vi "EnergyMonitoring.vi"() -> ()   [LabVIEW 2017]
uses:
  <vilib>/drjdpowell/SQLite Library/SQL Statement/SQL Statement.lvclass/SQL Statement.ctl
  <vilib>/drjdpowell/SQLite Library/SQL Connection/Open (path).vi
  <vilib>/drjdpowell/SQLite Library/SQL Statement/Column I64.vi
  <vilib>/drjdpowell/SQLite Library/SQL Statement/Column DBL.vi
  <vilib>/drjdpowell/SQLite Library/SQL Connection/Open (string).vi
  <vilib>/drjdpowell/SQLite Library/SQL Statement/Column Type.vi
  <vilib>/AdvancedString/Path To Command Line String.vi
  <vilib>/drjdpowell/SQLite Library/SQL Connection/Execute SQL.vi
  <vilib>/drjdpowell/SQLite Library/SQL Statement/Error Message.vi
  <vilib>/drjdpowell/SQLite Library/SQL Statement/Column Timestamp.vi
  <vilib>/drjdpowell/SQLite Library/SQL Statement/Column String.vi
  <vilib>/drjdpowell/SQLite Library/SQL Connection/Connection.lvclass
  <vilib>/drjdpowell/SQLite Library/SQL Statement/SQL Statement.lvclass
  <vilib>/drjdpowell/SQLite Library/SQLite.lvlib
panel:
  in  "Tab Control":enum32{"Monitor Values", "Monitor Diagram"}(tab)
  in  "Update":bool
  in  "Monitor Data of the Element":i32(listbox)=-1
  in  "Count of Points":i64(slide)=50 scale=0.0..100.0
  in  "x - Axis":u16(ring) items=["Index"]
  in  "y - Axis":i32(listbox)
  out "Graph":cluster{dbl[], dbl[]}(graph) caption="Selected data points (greater than \"minimum\")"
  in  "Update Trigger [sec]":i32=3
  in  "Count of Points Diagram":i64(slide)=50 scale=0.0..100.0
  out "Column:Get Column I64":i64
  in  "Field Elements":i32(listbox)
  in  "stop":bool
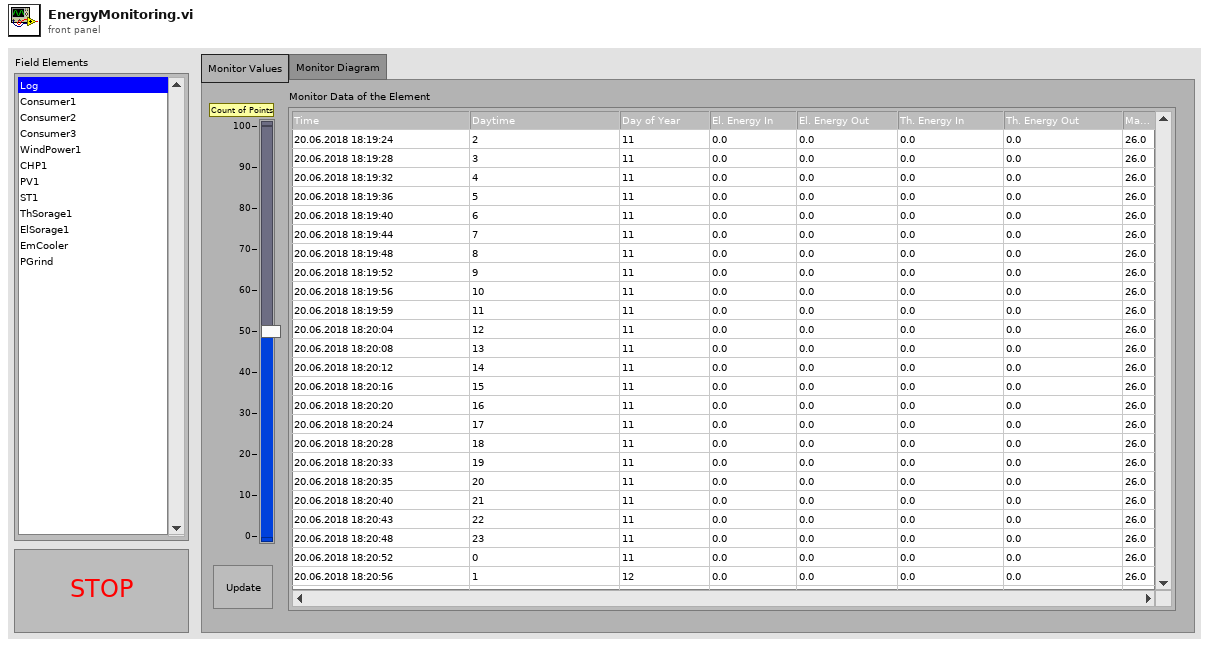
[diagram p1: front panel]
types:
  T1 = enum16{"New or existing", "Existing", "Read only"}
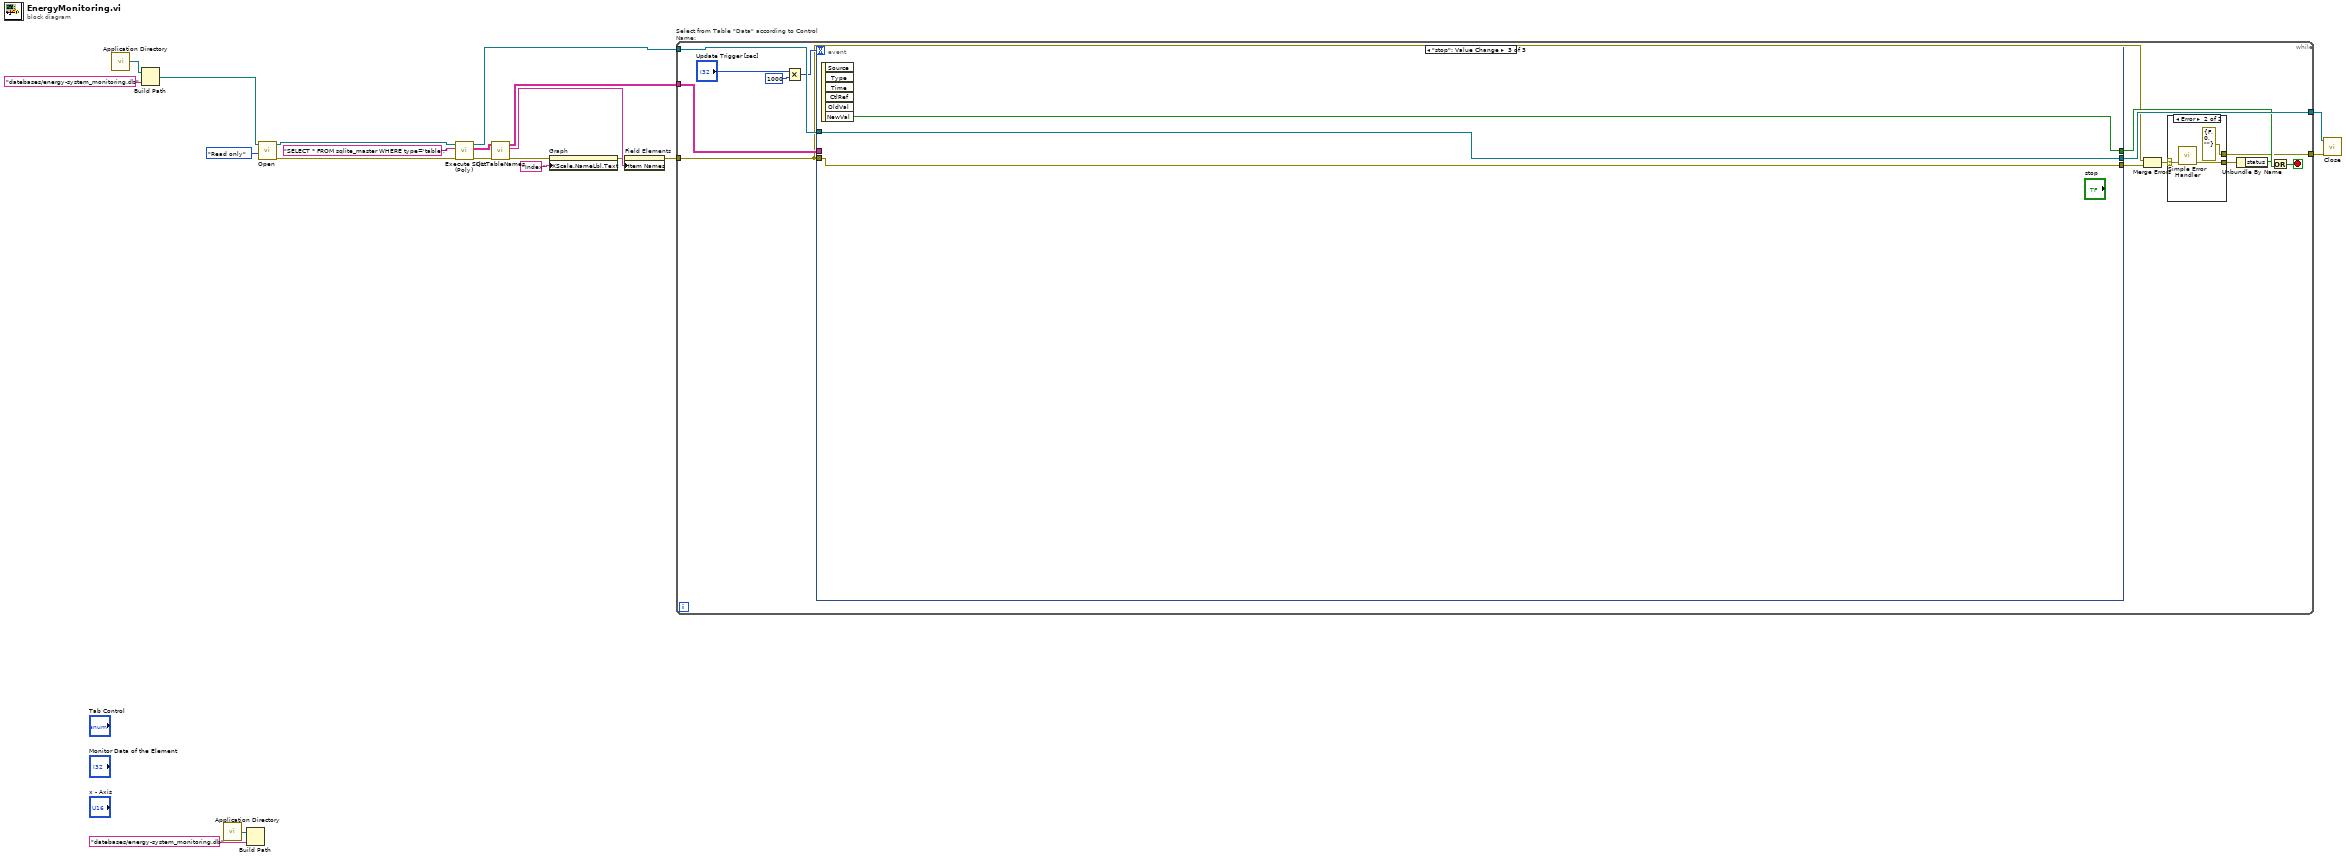
[diagram p0: block diagram]
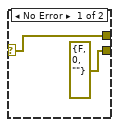
[diagram p2: hidden frame]
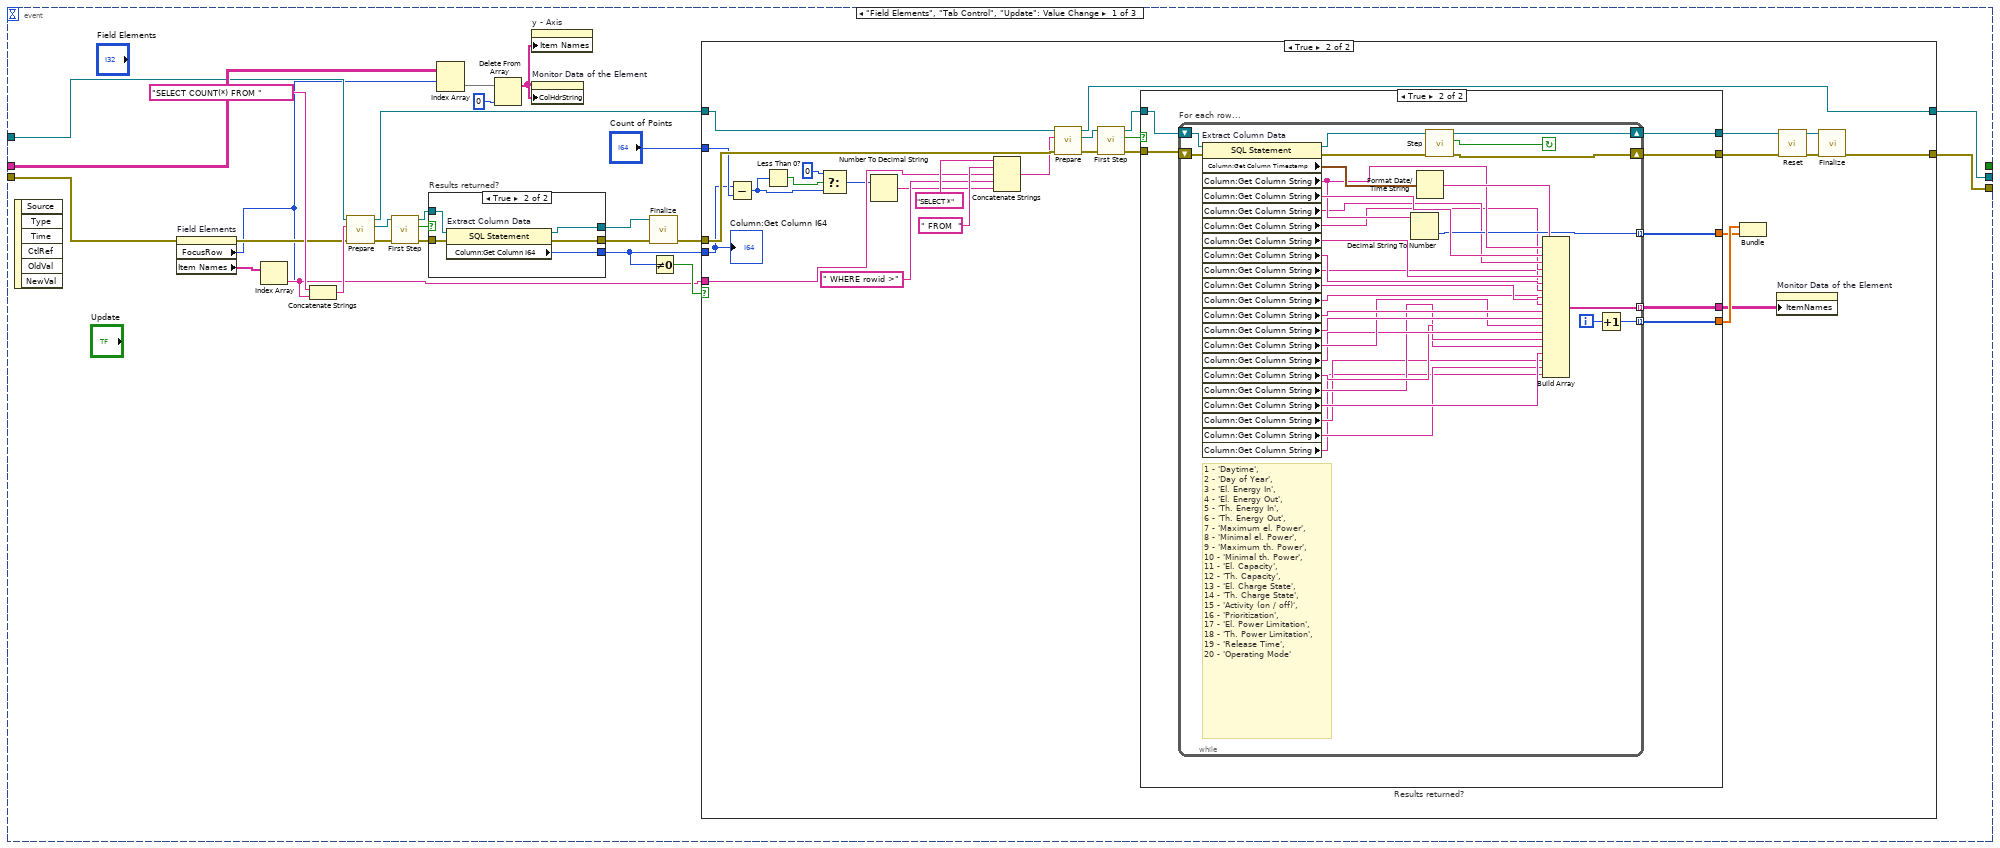
[diagram p3: hidden frame]
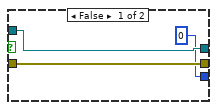
[diagram p4: hidden frame]
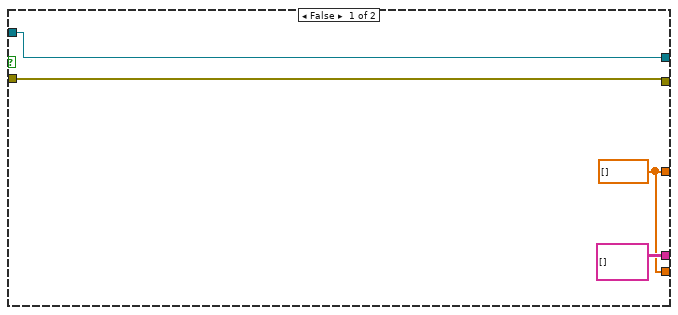
[diagram p6: hidden frame]
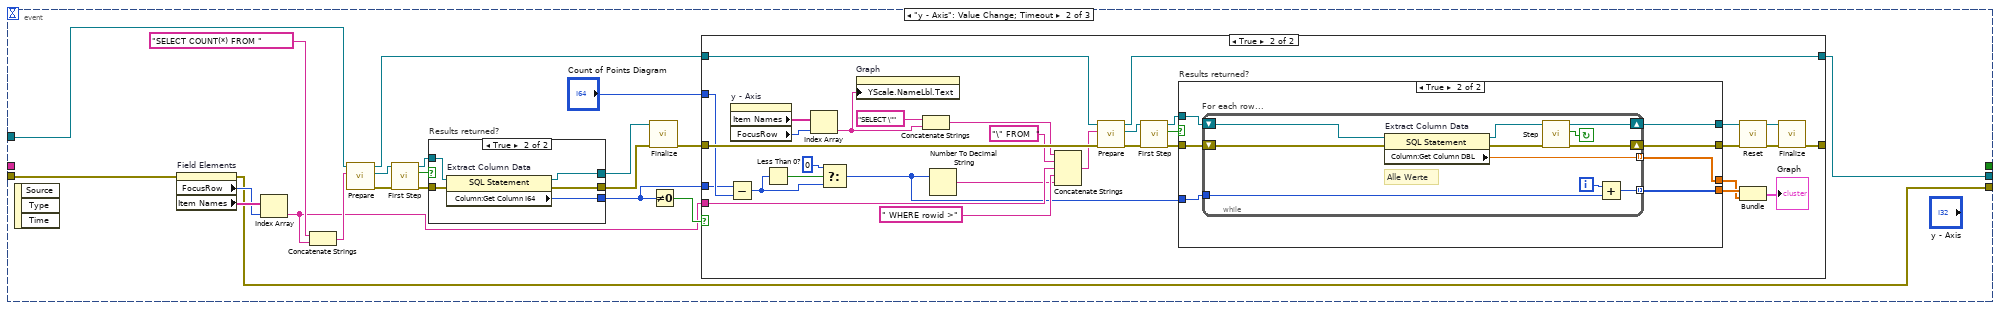
[diagram p7: hidden frame]
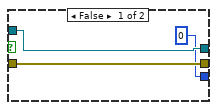
[diagram p8: hidden frame]
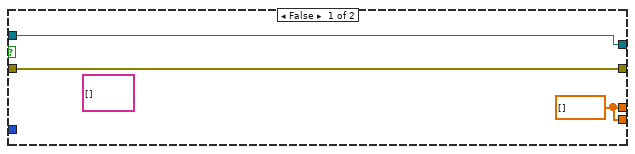
[diagram p10: hidden frame]
diagram:
  n1 = call <vilib>:"Application Directory.vi"() -> ("Application Directory"=w3:path)
  n2 = Build Path(base path=w3, name or relative path="datebases/energy-system_monitoring.db" ("Name oder relativer Pfad")) -> (appended path=w1:path)
  n3 = call <vilib>:"Application Directory.vi"() -> ("Application Directory"=w18:path)
  n4 = Build Path(base path=w18, name or relative path="datebases/energy-system_monitoring.db" ("Name oder relativer Pfad")) -> ()  [unwired: 1 out]
  n5 = call-poly <vilib>:"Open.vi"("File Option"=T1."Read only", "db file"=w1) -> ("error out"=w17:errorcluster, "SQLite Connection out"=w16:refnum<class "Connection.lvclass">)  [unwired: 8 in]
  n6 = call-poly <vilib>:"Execute SQL (Poly).vi"("error in (no error)"=w17, "SQL"="SELECT * FROM sqlite_master WHERE type='table';" ("String"), "SQLite Connection in"=w16) -> ("error out"=w6:errorcluster, "Result Set"=w10:string[][], "SQLite Connection out"=w14:refnum<class "Connection.lvclass">)  [unwired: 5 in, 1 out]
  n7 = call "ListTableNames.vi"("error in (no error)"=w6, "Result Set"=w10) -> ("error out"=w5:errorcluster, "Table Names"=w9:string[], "List of Tabel and Column Names"=w8:string[][])  [unwired: 7 in]
  n8 = property on="Graph" class="XYGraph (strict)"(error in=w5, "XScale.NameLbl.Text"="Index" ("X Scale.Name Label.Text")) -> (error out=w4:errorcluster)  [unwired: 1 in, 1 out]
  n9 = property on="Field Elements" class="LstBox (strict)"(error in=w4, "Item Names"=w9) -> (error out=w15:errorcluster)  [unwired: 1 in, 1 out]
  n10 = while "Select from Table \"Data\" according to Control Name:" {
    tunnel: [w24] -> w12
    tunnel: w15 -> [w23]
    tunnel: w14 -> [w34]
    tunnel: [w33] -> w13
    tunnel: w8 -> [w29]
    stop <- w27 stop-if-true
    n11 = Multiply(x="Update Trigger [sec]", y=1000) -> (x*y=w30:i32)
    n12 = event shown="[2] \"stop\": Value Change" {
      selector: _ -> [_ _ _]
      dyn-events: _ -> [_ _ _]
      timeout: w30 -> [_ _ _]
      tunnel: [_ _ w233] -> w28
      tunnel: [w41 w150 w232] -> w22
      tunnel: w23 -> [w64 w165 w232]
      tunnel: w34 -> [w43 w148 w231]
      tunnel: [w49 w147 w231] -> w33
      tunnel: w29 -> [w48 _ _]
      event "Field Elements", "Tab Control", "Update": Value Change {
        n13 = event-data() -> ()  [unwired: 1 in, 6 out]
        n14 = property on="Field Elements" class="LstBox (strict)"(error in=w64) -> (error out=w44:errorcluster, "FocusRow"=w40:i32, "Item Names"=w65:string[])  [unwired: 1 in, 1 out]
        n15 = Index Array(array=w65, index=w40) -> (element=w42:string)
        n16 = Concatenate Strings("SELECT COUNT(*) FROM " ("String"), w42) -> (w63:string)
        n17 = call <vilib>:"Prepare.vi"("error in (no error)"=w44, "SQL"=w63, "SQLite Connection in"=w43) -> ("error out"=w59:errorcluster, "SQL Statement out"=w58:refnum<class "SQL Statement.lvclass">, "SQLite Connection out"=w60:refnum<class "Connection.lvclass">)  [unwired: 4 in, 2 out]
        n18 = call <vilib>:"First Step.vi"("error in (no error)"=w59, "SQL Statement in"=w58) -> ("error out"=w57:errorcluster, "Row returned"=w55:bool, "SQL Statement out"=w56:refnum<class "SQL Statement.lvclass">)  [unwired: 7 in]
        n19 = case "Results returned?" shown="True" w55 {
          tunnel: [w68 w70] -> w53
          tunnel: [w67 w71] -> w54
          tunnel: w56 -> [w68 w73]
          tunnel: w57 -> [w67 w72]
          tunnel: [i64 0 ("Column:Get Column I64") w69] -> w61
          frame False {
          }
          frame True {
            n20 = property on="Extract Column Data" class="SQL Statement"(reference=w73, error in=w72) -> (reference out=w70:refnum<class "SQL Statement.lvclass">, error out=w71:errorcluster, "Column:Get Column I64"=w69:i64)
          }
        }
        n21 = Index Array(array=w48, index (row)=w40) -> (element=w45:string[])  [unwired: 1 in]
        n22 = Delete From Array(array=w45, index=0) -> (array with subset deleted=w46:string[])  [unwired: 1 in, 1 out]
        n23 = property on="y - Axis" class="LstBox (strict)"("Item Names"=w46) -> ()  [unwired: 2 in, 2 out]
        n24 = property on="Monitor Data of the Element" class="MCListbox (strict)"("ColHdrString"=w46) -> ()  [unwired: 2 in, 2 out]
        n25 = call <vilib>:"Finalize.vi"("error in (no error)"=w54, "SQL Statement in"=w53) -> ("error out"=w62:errorcluster)  [unwired: 9 in]
        n26 = Not Equal To 0?(x=w61) -> (x != 0?=w52:bool)
        n27 = case shown="True" w52 {
          tunnel: [w75 w83] -> w41
          tunnel: w60 -> [w74 w101]
          tunnel: w62 -> [w75 w100]
          tunnel: w61 -> [_ w89]
          tunnel: w42 -> [_ w97]
          tunnel: "Count of Points" -> [_ w91]
          tunnel: [w74 w81] -> w49
          frame False {
          }
          frame True {
            n28 = Subtract(x=w89, y=w91) -> (x-y=w80:i64)
            n29 = Less Than 0?(x=w80) -> (x < 0?=w90:bool)
            n30 = Select(t=i64 0 ("y"), s=w90, f=w80) -> (s? t:f=w87:i64)
            n31 = Number To Decimal String(number=w87) -> (decimal integer string=w88:string)  [unwired: 1 in]
            n32 = Concatenate Strings("SELECT *" ("string"), " FROM  " ("string"), w97, " WHERE rowid >" ("string"), w88) -> (w96:string)
            n33 = call <vilib>:"Prepare.vi"("error in (no error)"=w100, "SQL"=w96, "SQLite Connection in"=w101) -> ("error out"=w103:errorcluster, "SQL Statement out"=w102:refnum<class "SQL Statement.lvclass">, "SQLite Connection out"=w81:refnum<class "Connection.lvclass">)  [unwired: 4 in, 2 out]
            n34 = call <vilib>:"First Step.vi"("error in (no error)"=w103, "SQL Statement in"=w102) -> ("error out"=w94:errorcluster, "Row returned"=w92:bool, "SQL Statement out"=w93:refnum<class "SQL Statement.lvclass">)  [unwired: 7 in]
            n35 = case "Results returned?" shown="True" w92 {
              tunnel: [w107 w114] -> w85
              tunnel: [w106 w113] -> w86
              tunnel: w93 -> [w107 w112]
              tunnel: w94 -> [w106 w111]
              tunnel: [string[][] [] w110] -> w76
              tunnel: [w104 w109] -> w78
              tunnel: [w104 w108] -> w77
              frame False {
                w104 = dbl[] []
              }
              frame True {
                n36 = while "For each row..." {
                  shift-right: [w145] -> w114
                  shift-left: w112 -> [w142]
                  shift-right: [w143] -> w113
                  shift-left: w111 -> [w141]
                  tunnel: [w137] -> w110 mode=indexing
                  tunnel: [w134] -> w109 mode=indexing
                  tunnel: [w132] -> w108 mode=indexing
                  i -> [w135]
                  stop <- w140 continue-if-true
                  # "1 - 'Daytime', \n2 - 'Day of Year', \n3 - 'El. Energy In',  \n4 - 'El. Energy Out', \n5 - 'Th. Energy In',  \n6 - 'Th. Energy Out',  \n7 - 'Maximum el. Power', \n8 - 'Minimal el. Power', \n9 - 'Maximum th. Power', \n10 - 'Minimal th. Power', \n11 - 'El. Capacity',  \n12 - 'Th. Capacity',\n13 - 'El. Charge State', \n14 - 'Th. Charge State', \n15 - 'Activity (on / off)', \n16 - 'Prioritization', \n17 - 'El. Power Limitation',  \n18 - 'Th. Power Limitation',\n19 - 'Release Time',\n20 - 'Operating Mode'"
                  n37 = property on="Extract Column Data" class="SQL Statement"(reference=w142, error in=w141) -> (reference out=w146:refnum<class "SQL Statement.lvclass">, error out=w144:errorcluster, "Column:Get Column Timestamp"=w138:timestamp, "Column:Get Column String"=w133:string, "Column:Get Column String"=w136:string, "Column:Get Column String"=w131:string, "Column:Get Column String"=w130:string, "Column:Get Column String"=w129:string, "Column:Get Column String"=w128:string, "Column:Get Column String"=w127:string, "Column:Get Column String"=w126:string, "Column:Get Column String"=w125:string, "Column:Get Column String"=w124:string, "Column:Get Column String"=w123:string, "Column:Get Column String"=w122:string, "Column:Get Column String"=w121:string, "Column:Get Column String"=w120:string, "Column:Get Column String"=w119:string, "Column:Get Column String"=w118:string, "Column:Get Column String"=w117:string, "Column:Get Column String"=w116:string, "Column:Get Column String"=w115:string)
                  n38 = Decimal String To Number(string=w133) -> (number=w132:i32)  [unwired: 2 in, 1 out]
                  n39 = Format Date/Time String(seconds (now)=w138) -> (date/time string=w139:string)  [unwired: 2 in]
                  n40 = call <vilib>:"Step.vi"("error in (no error)"=w144, "SQL Statement in"=w146) -> ("error out"=w143:errorcluster, "Row returned"=w140:bool, "SQL Statement out"=w145:refnum<class "SQL Statement.lvclass">)  [unwired: 7 in]
                  n41 = Build Array(w139, w133, w136, w131, w130, w129, w128, w127, w126, w125, w124, w123, w122, w121, w120, w119, w118, w117, w116, w115) -> (w137:string[])
                  n42 = Increment(x=w135) -> (x+1=w134:i32)
                }
              }
            }
            n43 = Bundle(w78, w77) -> ()  [unwired: 1 in, 1 out]
            n44 = property on="Monitor Data of the Element" class="MCListbox (strict)"("ItemNames"=w76) -> ()  [unwired: 2 in, 2 out]
            n45 = call <vilib>:"Reset.vi"("error in (no error)"=w86, "SQL Statement in"=w85) -> ("error out"=w84:errorcluster, "SQL Statement out"=w82:refnum<class "SQL Statement.lvclass">)  [unwired: 8 in]
            n46 = call <vilib>:"Finalize.vi"("error in (no error)"=w84, "SQL Statement in"=w82) -> ("error out"=w83:errorcluster)  [unwired: 9 in]
            "Column:Get Column I64" <- w89
          }
        }
      }
      event "y - Axis": Value Change; Timeout {
        n47 = event-data() -> ()  [unwired: 1 in, 3 out]
        n48 = property on="Field Elements" class="LstBox (strict)"(error in=w165) -> (error out=w150:errorcluster, "FocusRow"=w166:i32, "Item Names"=w167:string[])  [unwired: 1 in, 1 out]
        n49 = Index Array(array=w167, index=w166) -> (element=w149:string)
        n50 = Concatenate Strings("SELECT COUNT(*) FROM " ("String"), w149) -> (w164:string)
        n51 = call <vilib>:"Prepare.vi"("SQL"=w164, "SQLite Connection in"=w148) -> ("error out"=w160:errorcluster, "SQL Statement out"=w159:refnum<class "SQL Statement.lvclass">, "SQLite Connection out"=w161:refnum<class "Connection.lvclass">)  [unwired: 5 in, 2 out]
        n52 = call <vilib>:"First Step.vi"("error in (no error)"=w160, "SQL Statement in"=w159) -> ("error out"=w158:errorcluster, "Row returned"=w156:bool, "SQL Statement out"=w157:refnum<class "SQL Statement.lvclass">)  [unwired: 7 in]
        n53 = case "Results returned?" shown="True" w156 {
          tunnel: [w170 w172] -> w154
          tunnel: [w169 w173] -> w155
          tunnel: w157 -> [w170 w175]
          tunnel: w158 -> [w169 w174]
          tunnel: [i64 0 ("Column:Get Column I64") w171] -> w162
          frame False {
          }
          frame True {
            n54 = property on="Extract Column Data" class="SQL Statement"(reference=w175, error in=w174) -> (reference out=w172:refnum<class "SQL Statement.lvclass">, error out=w173:errorcluster, "Column:Get Column I64"=w171:i64)
          }
        }
        n55 = call <vilib>:"Finalize.vi"("error in (no error)"=w155, "SQL Statement in"=w154) -> ("error out"=w163:errorcluster)  [unwired: 9 in]
        n56 = Not Equal To 0?(x=w162) -> (x != 0?=w153:bool)
        n57 = case shown="True" w153 {
          tunnel: [w177 w192] -> _
          tunnel: w161 -> [w176 w207]
          tunnel: w163 -> [w177 w206]
          tunnel: w162 -> [_ w180]
          tunnel: w149 -> [_ w204]
          tunnel: "Count of Points Diagram" -> [_ w198]
          tunnel: [w176 w190] -> w147
          frame False {
          }
          frame True {
            n58 = Subtract(x=w180, y=w198) -> (x-y=w189:i64)
            n59 = property on="y - Axis" class="LstBox (strict)"() -> ("Item Names"=w185:string[], "FocusRow"=w184:i32)  [unwired: 2 in, 2 out]
            n60 = Less Than 0?(x=w189) -> (x < 0?=w197:bool)
            n61 = Index Array(array=w185, index=w184) -> (element=w178:string)
            n62 = Select(t=i64 0 ("y"), s=w197, f=w189) -> (s? t:f=w179:i64)
            n63 = property on="Graph" class="XYGraph (strict)"("YScale.NameLbl.Text"=w178) -> ()  [unwired: 2 in, 2 out]
            n64 = Concatenate Strings("SELECT \"" ("string"), w178) -> (w182:string)
            n65 = Number To Decimal String(number=w179) -> (decimal integer string=w196:string)  [unwired: 1 in]
            n66 = Concatenate Strings(w182, "\" FROM  " ("string"), w204, " WHERE rowid >" ("string"), w196) -> (w203:string)
            n67 = call <vilib>:"Prepare.vi"("error in (no error)"=w206, "SQL"=w203, "SQLite Connection in"=w207) -> ("error out"=w209:errorcluster, "SQL Statement out"=w208:refnum<class "SQL Statement.lvclass">, "SQLite Connection out"=w190:refnum<class "Connection.lvclass">)  [unwired: 4 in, 2 out]
            n68 = call <vilib>:"First Step.vi"("error in (no error)"=w209, "SQL Statement in"=w208) -> ("error out"=w201:errorcluster, "Row returned"=w199:bool, "SQL Statement out"=w200:refnum<class "SQL Statement.lvclass">)  [unwired: 7 in]
            n69 = case "Results returned?" shown="True" w199 {
              tunnel: [w212 w219] -> w194
              tunnel: [w211 w218] -> w195
              tunnel: w200 -> [w212 w217]
              tunnel: w201 -> [w211 w216]
              tunnel: [w210 w215] -> w187
              tunnel: [w210 w214] -> w186
              tunnel: w179 -> [_ w213]
              frame False {
                w210 = dbl[] []
                (unwired) string[][] []
              }
              frame True {
                n70 = while "For each row..." {
                  shift-right: [w229] -> w219
                  shift-left: w217 -> [w226]
                  shift-right: [w227] -> w218
                  shift-left: w216 -> [w225]
                  tunnel: [w221] -> w215 mode=indexing
                  tunnel: [w220] -> w214 mode=indexing
                  tunnel: w213 -> [w222]
                  i -> [w223]
                  stop <- w224 continue-if-true
                  # "Alle Werte"
                  n71 = property on="Extract Column Data" class="SQL Statement"(reference=w226, error in=w225) -> (reference out=w230:refnum<class "SQL Statement.lvclass">, error out=w228:errorcluster, "Column:Get Column DBL"=w220:dbl)
                  n72 = call <vilib>:"Step.vi"("error in (no error)"=w228, "SQL Statement in"=w230) -> ("error out"=w227:errorcluster, "Row returned"=w224:bool, "SQL Statement out"=w229:refnum<class "SQL Statement.lvclass">)  [unwired: 7 in]
                  n73 = Add(x=w223, y=w222) -> (x+y=w221:i64)
                }
              }
            }
            n74 = call <vilib>:"Reset.vi"("error in (no error)"=w195, "SQL Statement in"=w194) -> ("error out"=w193:errorcluster, "SQL Statement out"=w191:refnum<class "SQL Statement.lvclass">)  [unwired: 8 in]
            n75 = Bundle(w187, w186) -> (→"Graph":cluster{dbl[], dbl[]})  [unwired: 1 in]
            n76 = call <vilib>:"Finalize.vi"("error in (no error)"=w193, "SQL Statement in"=w191) -> ("error out"=w192:errorcluster)  [unwired: 9 in]
          }
        }
      }
      event "stop": Value Change {
        n77 = event-data() -> ("NewVal"=w233:bool)  [unwired: 1 in, 5 out]
      }
    }
    n78 = Merge Errors(w23, w22) -> (w21:errorcluster)
    n79 = case shown="Error" w21 {
      selector: w21 -> [w35 w39]
      tunnel: [errorcluster {"status"=FALSE, "code"=0, "source"=""} ("error out") w38] -> w25
      tunnel: [w35 errorcluster {"status"=FALSE, "code"=0, "source"=""} ("error out")] -> w24
      frame No Error {
      }
      frame Error {
        n80 = call <vilib>:"Simple Error Handler.vi"("error in (no error)"=w39) -> ("error out"=w38:errorcluster)  [unwired: 4 in, 4 out]
      }
    }
    n81 = Unbundle By Name(w25) -> ("status"=w26:bool)
    n82 = Or(x=w26, y=w28) -> (x .or. y?=w27:bool)
  }
  n83 = call-dynamic "Close.vi"("error in (no error)"=w12, "SQLite Connection in"=w13) -> ()  [unwired: 9 in, 1 out]
